vi "i32_to_fxp.vi"(1 "32bit integer":i32) -> (0 "fxp32_16":fxp<+/-,32,16>)   [LabVIEW 2018]
uses:
  <vilib>/rvi/FXPMathLib/FxpInterpret/XNode/nifxpmath_Interpret.xnode
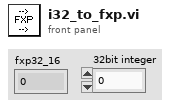
[diagram p1: front panel]
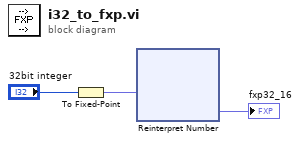
[diagram p0: block diagram]
diagram:
  n1 = To Fixed-Point(number="32bit integer") -> (fixed-point=w3:fxp<+/-,32,32>)  [unwired: 1 in]
  n2 = xnode "Reinterpret Number"("x"=w3) -> ("y"=→"fxp32_16":fxp<+/-,32,16>)
